vi "Warning Cluster Updater.vi"(1 "Warnings Cluster":T2) -> (0 "Warnings Cluster 2":T1)   [LabVIEW 2013]
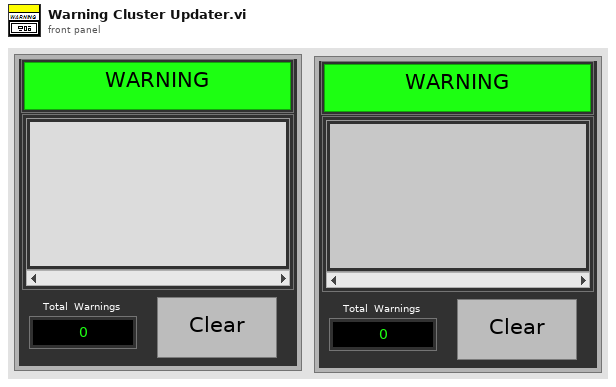
[diagram p1: front panel]
types:
  T1 = cluster{"Warning Array Out":string[], "Clear":bool, "Existing Warnings":i32[], "Num Warning Queue":i32[], "Total  Warnings":i32, "OK Button":bool, "Boolean":bool}
  T2 = cluster{"Warning Array Out":string[], "Clear":bool, "Existing Warnings":i32[], "Num Warning Queue":i32[], "Total  Warnings":i32, "OK Button":bool, "Warning Indicator":bool}
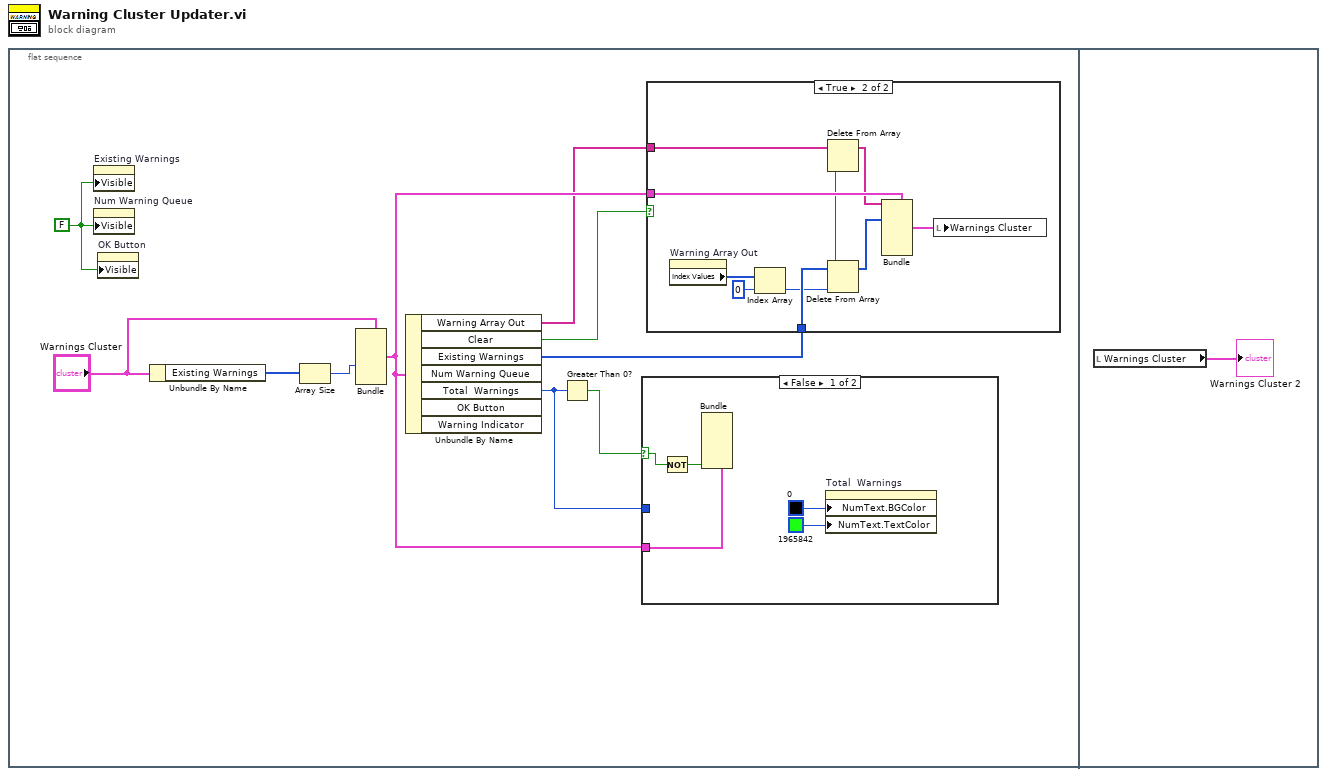
[diagram p0: block diagram]
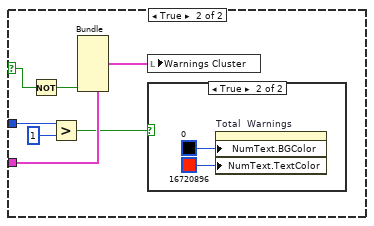
[diagram p3: hidden frame]
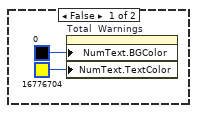
[diagram p4: hidden frame]
diagram:
  n1 = flat-sequence {
    frame #0 {
      w1 = FALSE ("Visible")
      n2 = property on="Existing Warnings" class="Arr (strict)"("Visible"=w1) -> ()  [unwired: 2 in, 2 out]
      n3 = property on="Num Warning Queue" class="Arr (strict)"("Visible"=w1) -> ()  [unwired: 2 in, 2 out]
      n4 = property on="OK Button" class="Bool (strict)"("Visible"=w1) -> ()  [unwired: 2 in, 2 out]
      n5 = Unbundle By Name("Warnings Cluster") -> ("Existing Warnings"=w10:i32[])
      n6 = Array Size(array=w10) -> (size(s)=w4:i32)
      n7 = Bundle(cluster="Warnings Cluster", "Total  Warnings"=w4) -> (w5:T2)  [unwired: 6 in]
      n8 = Unbundle By Name(w5) -> ("Warning Array Out"=w3:string[], "Clear"=w7:bool, "Existing Warnings"=w2:i32[], "Total  Warnings"=w6:i32)  [unwired: 3 out]
      n9 = Greater Than 0?(x=w6) -> (x > 0?=w8:bool)
      n10 = case shown="False" w8 {
        selector: w8 -> [w23 w30]
        tunnel: w5 -> [w24 w31]
        tunnel: w6 -> [_ w28]
        frame False {
          n11 = Not(x=w23) -> (.not. x?=w22:bool)
          n12 = Bundle(cluster=w24, "Warning Indicator"=w22) -> ()  [unwired: 6 in, 1 out]
          n13 = property on="Total  Warnings" class="DigNum (strict)"("NumText.BGColor"=u32 0, "NumText.TextColor"=u32 1965842) -> ()  [unwired: 2 in, 2 out]
        }
        frame True {
          n14 = Not(x=w30) -> (.not. x?=w29:bool)
          n15 = Greater?(x=w28, y=1) -> (0:w26:bool)
          n16 = Bundle(cluster=w31, "Warning Indicator"=w29) -> (w25:T2)  [unwired: 6 in]
          n17 = local write "Warnings Cluster"(w25) -> ()
          n18 = case shown="True" w26 {
            frame False {
              n19 = property on="Total  Warnings" class="DigNum (strict)"("NumText.BGColor"=u32 0, "NumText.TextColor"=u32 16776704) -> ()  [unwired: 2 in, 2 out]
            }
            frame True {
              n20 = property on="Total  Warnings" class="DigNum (strict)"("NumText.BGColor"=u32 0, "NumText.TextColor"=u32 16720896) -> ()  [unwired: 2 in, 2 out]
            }
          }
        }
      }
      n21 = case shown="True" w7 {
        tunnel: w5 -> [_ w19]
        tunnel: w3 -> [_ w17]
        tunnel: w2 -> [_ w16]
        frame False {
        }
        frame True {
          n22 = property on="Warning Array Out" class="Arr (strict)"() -> ("Index Values"=w14:u32[])  [unwired: 2 in, 2 out]
          n23 = Index Array(array=w14, index=0) -> (element=w13:u32)
          n24 = Delete From Array(array=w17, index=w13) -> (array with subset deleted=w12:string[])  [unwired: 1 in, 1 out]
          n25 = Delete From Array(array=w16, index=w13) -> (array with subset deleted=w11:i32[])  [unwired: 1 in, 1 out]
          n26 = Bundle(cluster=w19, "Warning Array Out"=w12, "Existing Warnings"=w11) -> (w18:T2)  [unwired: 5 in]
          n27 = local write "Warnings Cluster"(w18) -> ()
        }
      }
    }
    frame #1 {
      n28 = local read "Warnings Cluster"() -> (→"Warnings Cluster 2":T2)
    }
  }
